vi "Audio Playback Example.vi"() -> ()   [LabVIEW 2020]
doc: "Simple example of audio device playback of a file decoded with G-Audio."
uses:
  Controls/Audio Device Config.ctl
  Controls/Audio Device Format.ctl
  8289e2ef-86ba-4438-8a42-485f00fd8c95.vi
  9545a255-db38-479b-bcdc-619f4ee8d9ed.vi
  Private/Get Basic Audio File Info.vi
  Private/Result To Error.vi
  8289e2ef-86ba-4438-8a42-485f00fd8c95.vi/779dfdfd-1b42-4cf4-8001-66d3dd167625.vi
  8289e2ef-86ba-4438-8a42-485f00fd8c95.vi/55d550d4-9624-414e-aebd-6e02b5081896.vi
  Private/Audio File Refnum To Value.vi
  9545a255-db38-479b-bcdc-619f4ee8d9ed.vi/4dfb5711-8d81-45a3-b3db-a84d40650863.vi
  9545a255-db38-479b-bcdc-619f4ee8d9ed.vi/c8869513-30c6-44f2-a2d3-73232fe63870.vi
  Private/Audio Device Refnum To Value.vi
  8289e2ef-86ba-4438-8a42-485f00fd8c95.vi/55d550d4-9624-414e-aebd-6e02b5081896.vi/4b7b629c-2e91-4160-9820-a26af8f6e677.vi
  9545a255-db38-479b-bcdc-619f4ee8d9ed.vi/4dfb5711-8d81-45a3-b3db-a84d40650863.vi/4b7b629c-2e91-4160-9820-a26af8f6e677.vi
  9545a255-db38-479b-bcdc-619f4ee8d9ed.vi/c8869513-30c6-44f2-a2d3-73232fe63870.vi/4b7b629c-2e91-4160-9820-a26af8f6e677.vi
  Audio Files/Polymorphic VIs/Get Audio File Info (Path).vi
  Audio Files/Polymorphic VIs/Open Audio File Read (Path).vi
  <vilib>/Utility/Data Type/Get Numeric Information.vi
  <vilib>/Utility/error.llb/Error Cluster From Error Code.vi
  G-Audio.lvlib
panel:
  in  "Volume":sgl(slide)=1.0 min=0 max=1 step=0.01 scale=0.0..1.0
  out "Waveform":waveform(i16)[](graph)
  out "Now Playing:":string
  out "Duration":string
  out "Sample Length":u64
  out "Audio Info":T1
  out "error out":errorcluster
  in  "Stop":bool
  # "Instructions:\n1. Run the VI.\n2. Select an audio file to play.\n3. The VI will stop when the file has finished playing, or when the Stop button is pressed."
  # "G"
  # "-Audio"
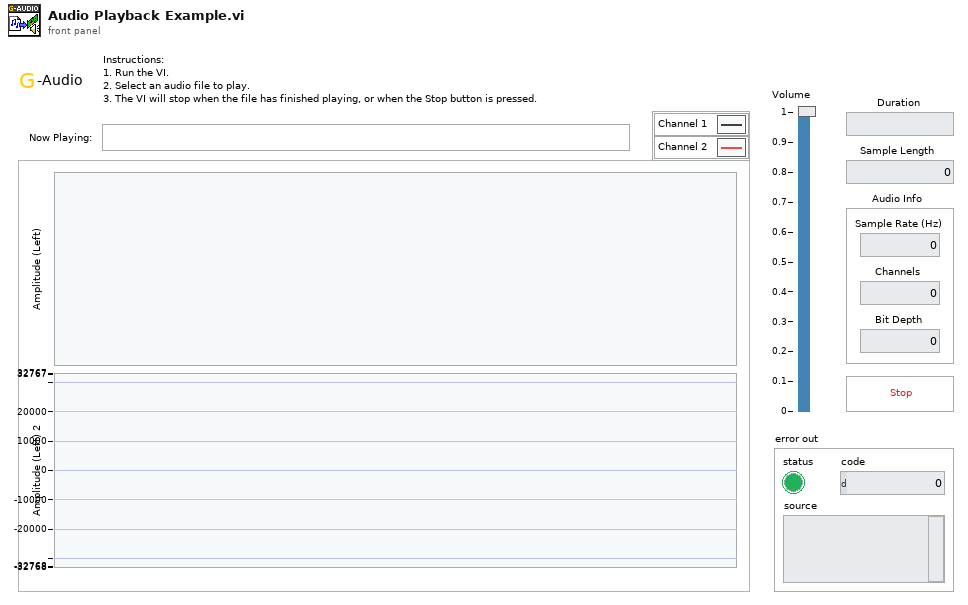
[diagram p1: front panel]
types:
  T1 = cluster{"Sample Rate (Hz)":u32, "Channels":u32, "Bit Depth":u32}
  T2 = typedef "G-Audio.lvlib/Audio Device Config.ctl" = cluster{"Sample Rate (Hz)":u32, "Channels":u32, "Format":T3}
  T3 = typedef "G-Audio.lvlib/Audio Device Format.ctl" = enum16{"Native", "U8", "I16", "I32", "SGL"}
  T4 = typedef "G-Audio.lvlib/Audio File Info.ctl" = cluster{"Sample Rate (Hz)":u32, "Channels":u32, "Bit Depth":u32}
  T5 = typedef "G-Audio.lvlib/Audio File Refnum.ctl" = refnum<file>
  T6 = typedef "G-Audio.lvlib/Audio Device Refnum.ctl" = refnum<file>
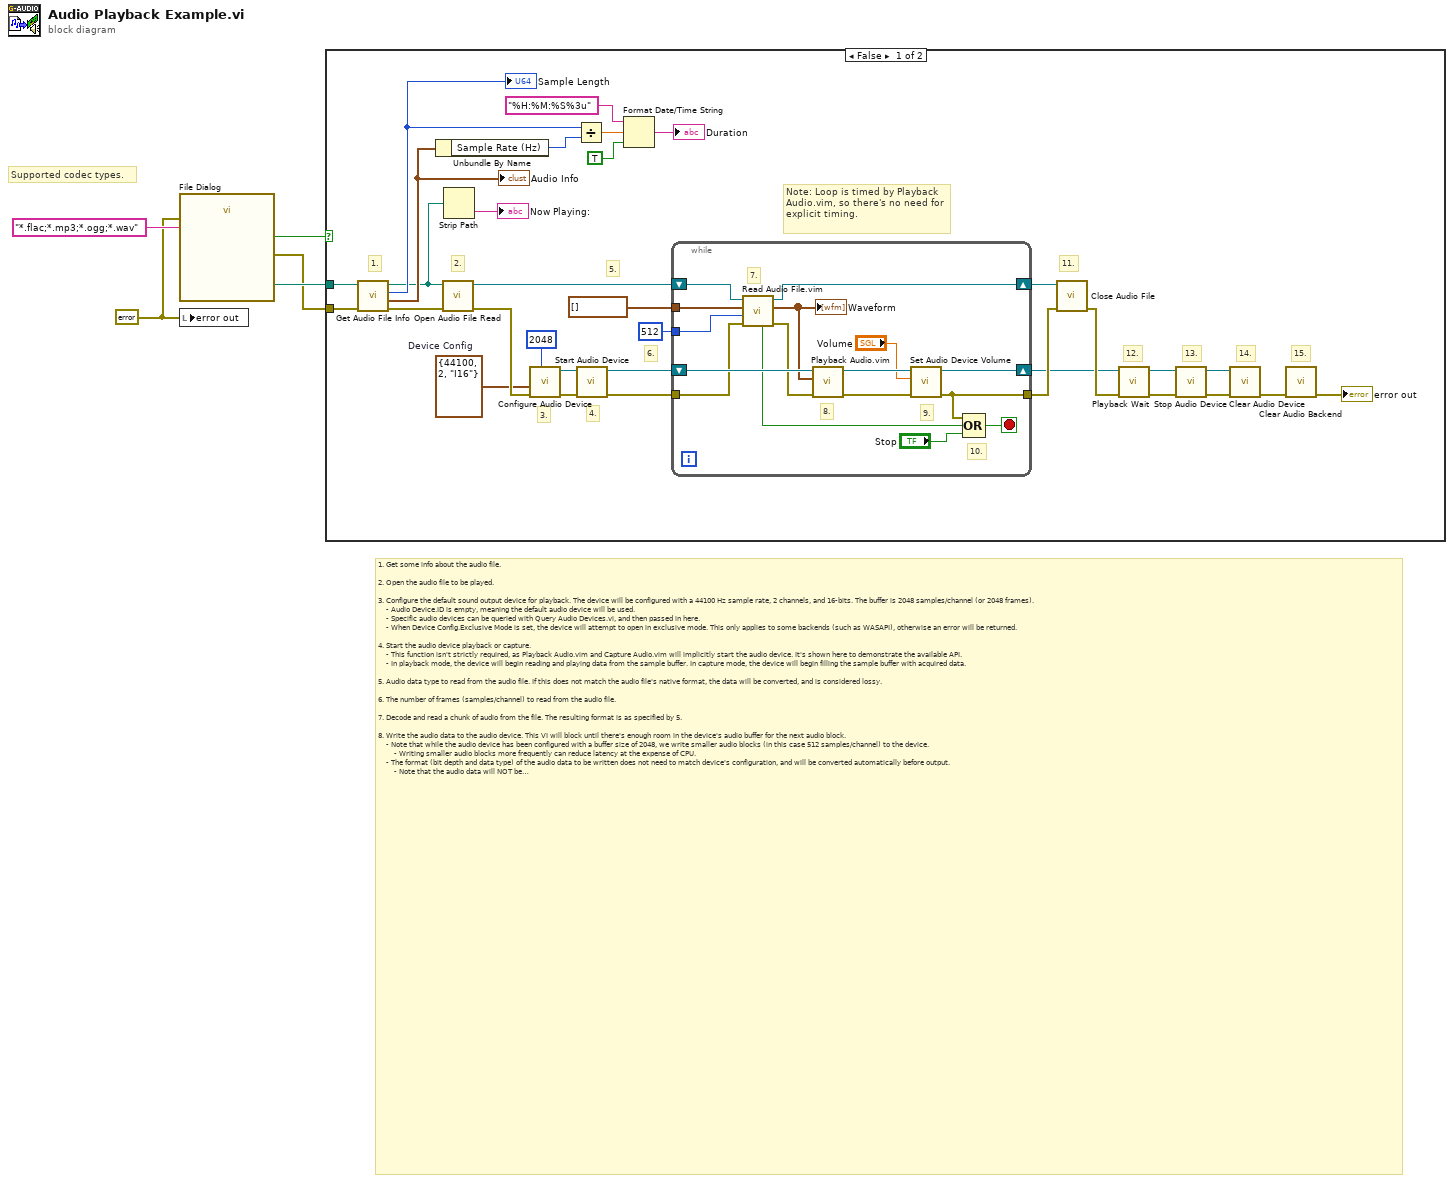
[diagram p0: block diagram]
diagram:
  w1 = errorcluster {"status"=FALSE, "code"=0, "source"=""} ("error out")
  # "1. Get some info about the audio file.\n\n2. Open the audio file to be played.\n\n3. Configure the default sound output device for playback. The device will be configured with a 44100 Hz sample rate, 2 channels, and 16-bits. The buffer is 2048 samples/channel (or 2048 frames).\n    - Audio Device.ID is empty, meaning the default audio device will be used.\n    - Specific audio devices can be queried with Query Audio Devices.vi, and then passed in here.\n    - When Device Config.Exclusive Mode is set, the device will attempt to open in exclusive mode. This only applies to some backends (such as WASAPI), otherwise an error will be returned.\n\n4. Start the audio device playback or capture.\n    - This function isn't strictly required, as Playback Audio.vim and Capture Audio.vim will implicitly start the audio device. It's shown here to demonstrate the available API.\n    - In playback mode, the device will begin reading and playing data from the sample buffer. In capture mode, the device will begin filling the sample buffer with acquired data.\n\n5. Audio data type to read from the audio file. If this does not match the audio file's native format, the data will be converted, and is considered lossy.\n\n6. The number of frames (samples/channel) to read from the audio file.\n\n7. Decode and read a chunk of audio from the file. The resulting format is as specified by 5.\n\n8. Write the audio data to the audio device. This VI will block until there's enough room in the device's audio buffer for the next audio block.\n    - Note that while the audio device has been configured with a buffer size of 2048, we write smaller audio blocks (in this case 512 samples/channel) to the device.\n        - Writing smaller audio blocks more frequently can reduce latency at the expense of CPU.\n    - The format (bit depth and data type) of the audio data to be written does not need to match device's configuration, and will be converted automatically before output.\n        - Note that the audio data will NOT be resampled.\n\n9. Set the audio device playback volume.\n\n10. Stop the loop when the end of file is reached, there's an error, or Stop was clicked.\n\n11. Close and cleanup the audio decoder.\n\n12. Wait for the audio device to finishing playing the content of the audio buffer.\n\n13. Stop the audio device.\n    - This function isn't strictly required, as Clear Audio Device.vi will implicitly stop the audio device. It's shown here to demonstrate the available API.\n    - Stopping the device does not clear or reset the audio buffer. If it is started again with Start Audio Device.vi, playback will resume.\n\n14. Clear the device and audio buffer. The device will become invalid.\n\n15. Clear the audio backend.\n    - Clearing the backend will forcibly stop all audio devices configured on that backend. It's only necessary to clear the backend if you wish to switch to another backend."
  # "Supported codec types."
  n1 = call "File Dialog"("error in"=w1, "pattern (all files)"="*.flac;*.mp3;*.ogg;*.wav") -> ("selected path"=w4:path, "cancelled"=w3:bool, "error out"=w2:errorcluster)  [unwired: 10 in, 1 out]
  n2 = local write "error out"(w1) -> ()
  n3 = case shown="False" w3 {
    tunnel: w4 -> [w8 _]
    tunnel: w2 -> [w37 _]
    frame False {
      w11 = T2 {"Sample Rate (Hz)"=44100, "Channels"=2, "Format"=enum."I16"}  # Device Config
      # "15."
      # "14."
      # "13."
      # "12."
      # "11."
      # "6."
      # "4."
      # "Note: Loop is timed by Playback Audio.vim, so there's no need for explicit timing."
      # "5."
      # "3."
      # "2."
      # "1."
      n4 = call-poly "Get Audio File Info.vi"("error in (no error)"=w37, "Path In"=w8) -> ("error out"=w36:errorcluster, "Audio File Info"=w24:T4, "PCM Frame Length"=w25:u64, "Path Out"=w7:path)  [unwired: 5 in, 1 out]
      "Audio Info" <- w24
      "Sample Length" <- w25
      n5 = Unbundle By Name(w24) -> ("Sample Rate (Hz)"=w23:u32)
      n6 = call-poly "Open Audio File Read.vi"("error in (no error)"=w36, "Path"=w7) -> ("error out"=w12:errorcluster, "Audio File Refnum"=w27:T5)  [unwired: 8 in]
      n7 = Strip Path(path=w7) -> (name=→"Now Playing:":string)  [unwired: 1 out]
      n8 = call "Configure Audio Device.vi"("Buffer Size (4096)"=2048 ("number of samples/ch"), "error in (no error)"=w12, "Device Config"=w11) -> ("error out"=w18:errorcluster, "Audio Device Refnum"=w17:T6)  [unwired: 5 in, 2 out]
      n9 = Divide(x=w25, y=w23) -> (x/y=w22:dbl)
      n10 = call "Start Audio Device.vi"("error in (no error)"=w18, "Audio Device Refnum In"=w17) -> ("error out"=w29:errorcluster, "Audio Device Refnum Out"=w30:T6)  [unwired: 8 in]
      n11 = Format Date/Time String(time format string (%c)="%H:%M:%S%3u", seconds (now)=w22, UTC format=TRUE) -> (date/time string=→"Duration":string)
      n12 = while {
        shift-right: [w51] -> w35
        shift-left: w27 -> [w53]
        shift-right: [w41] -> w14
        shift-left: w30 -> [w52]
        tunnel: w29 -> [w50]
        tunnel: [w38] -> w33
        tunnel: u64 512 ("number of samples/ch") -> [w45]
        tunnel: waveform(i16)[] [] -> [w44]
        stop <- w47 stop-if-true
        # "10."
        # "9."
        # "8."
        # "7."
        n13 = call "Read Audio File.vim"("error in (no error)"=w50, "Frames To Read"=w45, "Data Format"=w44, "Audio File Refnum In"=w53) -> ("error out"=w49:errorcluster, "Audio Data"=w43:waveform(i16)[], "Audio File Refnum Out"=w51:T5, "End of File?"=w48:bool)  [unwired: 3 in, 1 out]
        "Waveform" <- w43
        n14 = call "Playback Audio.vim"("error in (no error)"=w49, "Audio Data"=w43, "Audio Device Refnum In"=w52) -> ("error out"=w39:errorcluster, "Audio Device Refnum Out"=w42:T6)  [unwired: 7 in]
        n15 = call "Set Audio Device Volume.vi"("error in (no error)"=w39, "Volume"="Volume", "Audio Device Refnum In"=w42) -> ("error out"=w38:errorcluster, "Audio Device Refnum Out"=w41:T6)  [unwired: 7 in]
        n16 = Compound Arithmetic op=OR(w38, w48, "Stop") -> (w47:bool)
      }
      n17 = call "Close Audio File.vi"("error in (no error)"=w33, "Audio File Refnum In"=w35) -> ("error out"=w32:errorcluster)  [unwired: 9 in]
      n18 = call "Playback Wait.vi"("error in (no error)"=w32, "Audio Device Refnum In"=w14) -> ("error out"=w15:errorcluster, "Audio Device Refnum Out"=w13:T6)  [unwired: 8 in]
      n19 = call "Stop Audio Device.vi"("error in (no error)"=w15, "Audio Device Refnum In"=w13) -> ("error out"=w31:errorcluster, "Audio Device Refnum Out"=w34:T6)  [unwired: 8 in]
      n20 = call "Clear Audio Device.vi"("error in (no error)"=w31, "Audio Device Refnum In"=w34) -> ("error out"=w28:errorcluster)  [unwired: 9 in]
      n21 = call "Clear Audio Backend.vi"("error in (no error)"=w28) -> ("error out"=→"error out":errorcluster)  [unwired: 10 in]
    }
    frame True {
    }
  }
